vi "Hi_Tec_Comms.vi"(0 "Ch Description Array":T1[](array[typedef]) {"Duty" format="%.0b"; "D" format="%#_5g"; "C" format="%#_5g"; "B" format="%#_5g"; "A" format="%#_5g"}, 1 "Type":enum16{"Carrier", "Trace"}(ring), 2 "Hi Tec's To Change":bool[](array[boolean]), 3 "Client Name":string, 4 "Dem Volts":dbl[](array[numeric])) -> (5 "Outputs":dbl[](array[numeric]) format="%.2f")   [LabVIEW 2014]
uses:
  ADAM Client/Sub VIs/ADAM Controls/Ch_description_ADAM.ctl
  ADAM Client/Sub VIs/ADAM Controls/Module_type_ADAM.ctl
  ADAM Client/Sub VIs/ADAM Controls/Function_ADAM.ctl
  ADAM Client/Sub VIs/ADAM Controls/Channel_State.ctl
  ADAM Client/Sub VIs/ADAM Controls/Calib_type_ADAM.ctl
  ADAM Client/Sub VIs/ADAM Controls/Address.ctl
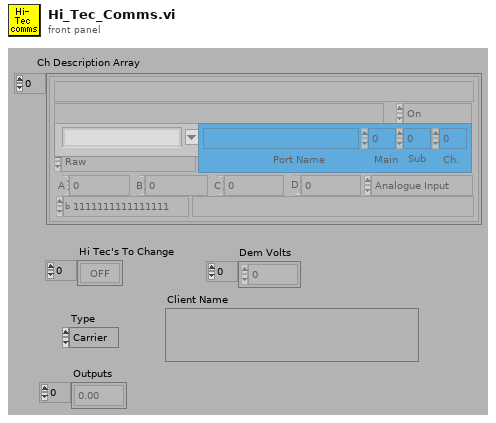
[diagram p1: front panel]
types:
  T1 = typedef "Ch_description_ADAM.ctl" = cluster{"Ch Name":string, "Type":T2, "Function":T3, "Ch State":T4, "Calibration type":T5, "A":dbl, "B":dbl, "C":dbl, "D":dbl, "Comments":string, "Address":T6, "String":string, "Duty":u16}
  T2 = typedef "Module_type_ADAM.ctl" = string
  T3 = typedef "Function_ADAM.ctl" = enum16{"Analogue Input", "Digital Input", "Event counter", "Event rate", "Analogue Output", "Digital Output", "Relay Output"}
  T4 = typedef "Channel_State.ctl" = enum16{"On", "Off", "Always On", "Always Off"}
  T5 = typedef "Calib_type_ADAM.ctl" = enum16{"Raw", "Bx + A", "Cx^2 + Bx + A", "Dx^3 + Cx^2 + Bx + A", "In Band", "Hi-Tec Q", "Hi-Tec M_dot", "Text"}
  T6 = typedef "Address.ctl" = cluster{"Main":i32, "Ch.":i32, "Sub":i32, "Port Name":string}
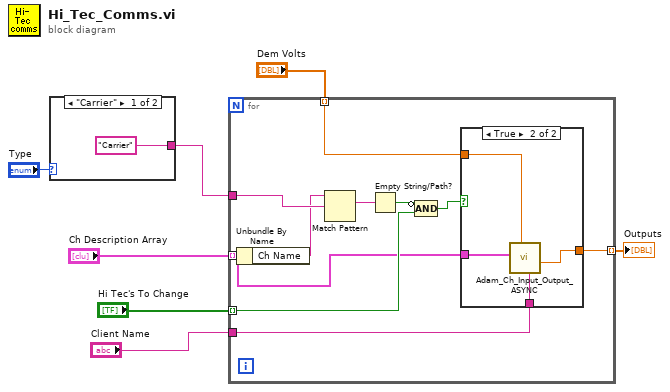
[diagram p0: block diagram]
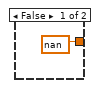
[diagram p2: hidden frame]
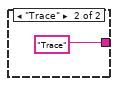
[diagram p3: hidden frame]
diagram:
  n1 = case shown="\"Carrier\"" "Type" {
    tunnel: ["Carrier" "Trace"] -> w6
    frame "Carrier" {
    }
    frame "Trace" {
    }
  }
  n2 = for {
    tunnel: w6 -> [w19]
    tunnel: "Ch Description Array" -> [w13] mode=indexing
    tunnel: "Hi Tec's To Change" -> [w14] mode=indexing
    tunnel: [w12] -> w3 mode=indexing
    tunnel: "Client Name" -> [w11]
    tunnel: "Dem Volts" -> [w10] mode=indexing
    n3 = Unbundle By Name(w13) -> ("Ch Name"=w18:string)
    n4 = Match Pattern(string=w18, regular expression=w19) -> (match substring=w17:string)  [unwired: 4 out]
    n5 = Empty String/Path?(string/path=w17) -> (empty?=w16:bool)
    n6 = Compound Arithmetic op=AND(invert w16, w14) -> (w15:bool)
    n7 = case shown="True" w15 {
      tunnel: w13 -> [_ w24]
      tunnel: [nan w23] -> w12
      tunnel: w11 -> [_ w22]
      tunnel: w10 -> [_ w21]
      frame False {
      }
      frame True {
        n8 = call "Adam_Ch_Input_Output_ASYNC.vi"("Client Name"=w22, "Value to Output"=w21, "Ch Discription"=w24) -> ("Calibrated units"=w23:dbl)  [unwired: 4 in, 4 out]
      }
    }
  }
  "Outputs" <- w3
